vi "Start or Stop Terminals.vi"(6 "trigger values":dbl[](array[numeric]), 7 "minor frame period (us)":i32, 8 "error in":errorcluster, 9 "running status":T1[](array[typedef]), 10 "terminal addresses":T3[](array[typedef]), 11 "module reference":T2) -> (0 "error out":errorcluster, 1 "running status out":T1[](array[typedef]))   [LabVIEW 2020, in "AIM MIL-STD-1553 Engine.lvlib" / "Implementation.lvlib" / "Triggers Execution Unit.lvclass"]
uses:
  Triggers Execution Unit.lvclass
  Shared/Address.ctl
  Hardware API/Module Reference.ctl
  Shared/Running Status.ctl
  Hardware API/AIM MIL-STD-1553 Hardware API.lvlib
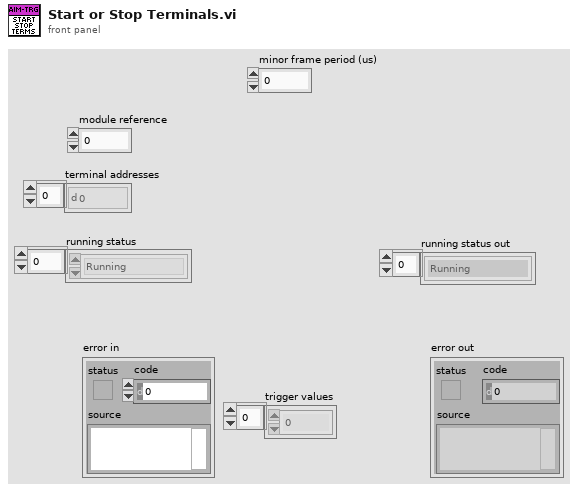
[diagram p1: front panel]
types:
  T1 = typedef "Running Status.ctl" = enum16{"Running", "Stopped"}
  T2 = typedef "AIM MIL-STD-1553 Hardware API.lvlib/Module Reference.ctl" = u32
  T3 = typedef "Address.ctl" = u16
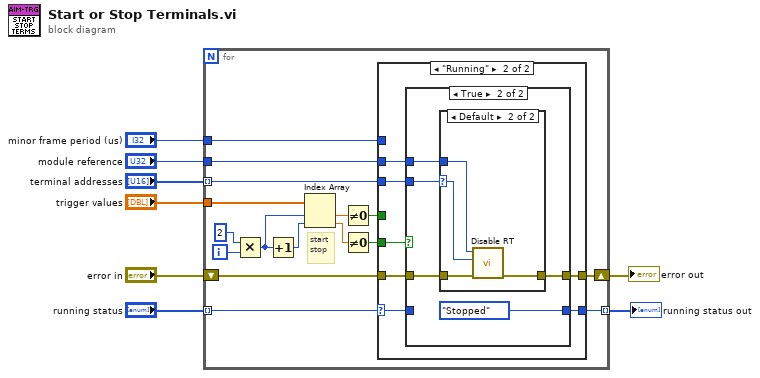
[diagram p0: block diagram]
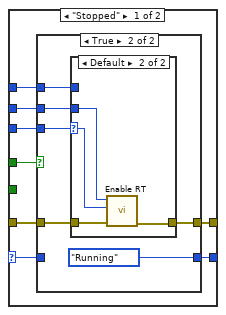
[diagram p2: hidden frame]
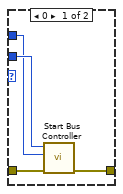
[diagram p4: hidden frame]
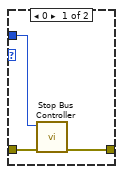
[diagram p6: hidden frame]
diagram:
  n1 = for {
    tunnel: "terminal addresses" -> [w15] mode=indexing
    tunnel: "module reference" -> [w10]
    tunnel: "running status" -> [w9] mode=indexing
    tunnel: "trigger values" -> [w22]
    shift-right: [w13] -> w3
    shift-left: "error in" -> [w14]
    tunnel: "minor frame period (us)" -> [w12]
    tunnel: [w11] -> w1 mode=indexing
    i -> [w24]
    # "start\nstop"
    n2 = Multiply(x=2, y=w24) -> (x*y=w21:i32)
    n3 = Increment(x=w21) -> (x+1=w20:i32)
    n4 = Index Array(array=w22, index #1=w21, index #2=w20) -> (element #1=w18:dbl, element #2=w19:dbl)
    n5 = Not Equal To 0?(x=w18) -> (x != 0?=w17:bool)
    n6 = Not Equal To 0?(x=w19) -> (x != 0?=w16:bool)
    n7 = case shown="\"Running\"" w9 {
      selector: w9 -> [w27 w52]
      tunnel: w17 -> [w31 _]
      tunnel: w16 -> [_ w49]
      tunnel: w15 -> [w32 w55]
      tunnel: w14 -> [w30 w54]
      tunnel: [w29 w53] -> w13
      tunnel: w12 -> [w28 _]
      tunnel: [w26 w51] -> w11
      tunnel: w10 -> [w25 w50]
      frame "Stopped" {
        n8 = case shown="True" w31 {
          tunnel: w32 -> [_ w40]
          tunnel: w30 -> [w34 w39]
          tunnel: [w34 w38] -> w29
          tunnel: w28 -> [_ w37]
          tunnel: w27 -> [w33 _]
          tunnel: [w33 Running_Status."Running" ("Running Status")] -> w26
          tunnel: w25 -> [_ w35]
          frame False {
          }
          frame True {
            n9 = case shown="Default" w40 {
              selector: w40 -> [_ w46]
              tunnel: w39 -> [w44 w48]
              tunnel: [w43 w47] -> w38
              tunnel: w37 -> [w41 _]
              tunnel: w35 -> [w42 w45]
              frame 0 {
                n10 = call "Start Bus Controller.vi"("error in"=w44, "minor frame period (us)"=w41, "module handle"=w42) -> ("error out"=w43:errorcluster)  [unwired: 7 in, 1 out]
              }
              frame Default {
                n11 = call "Enable RT.vi"("error in"=w48, "terminal address"=w46, "module handle"=w45) -> ("error out"=w47:errorcluster)  [unwired: 7 in, 1 out]
              }
            }
          }
        }
      }
      frame "Running" {
        n12 = case shown="True" w49 {
          tunnel: w55 -> [_ w62]
          tunnel: w54 -> [w57 w61]
          tunnel: [w57 w60] -> w53
          tunnel: w52 -> [w56 _]
          tunnel: [w56 Running_Status."Stopped" ("Running Status")] -> w51
          tunnel: w50 -> [_ w58]
          frame False {
          }
          frame True {
            n13 = case shown="Default" w62 {
              selector: w62 -> [_ w66]
              tunnel: w61 -> [w65 w69]
              tunnel: [w64 w68] -> w60
              tunnel: w58 -> [w63 w67]
              frame 0 {
                n14 = call "Stop Bus Controller.vi"("error in"=w65, "module handle"=w63) -> ("error out"=w64:errorcluster)  [unwired: 8 in, 1 out]
              }
              frame Default {
                n15 = call "Disable RT.vi"("error in"=w69, "terminal address"=w66, "module handle"=w67) -> ("error out"=w68:errorcluster)  [unwired: 7 in, 1 out]
              }
            }
          }
        }
      }
    }
  }
  "error out" <- w3
  "running status out" <- w1
